vi "Inverse Kinematics Solution to Pod Setpoints.vi"(10 "actual theta":dbl, 11 "v + target":cluster{"velocity":dbl, "target theta":dbl}) -> (3 "new v + travel":cluster{"velocity":dbl, "travel angle":dbl})   [LabVIEW 2020]
doc: "takes the <b>current velocity</b> and <b>wanted target angle</b> to travel, finds the most efficient angle to travel, and outputs the <b>new velocity</b> and the <b>travel angle.</b>\n(used in inverse kinematics)"
uses:
  <vilib>/Analysis/coordinate.llb/Angle Units.ctl
  <vilib>/Analysis/coordinate.llb/Angle Range (Degree).ctl
  <vilib>/Analysis/coordinate.llb/Wrap Angle (scalar).vi
  <vilib>/Analysis/NI_AAL_Angle.lvlib
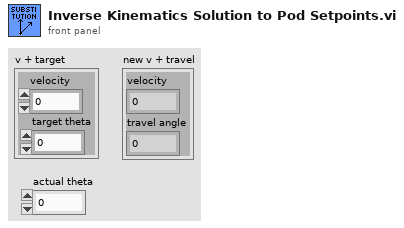
[diagram p1: front panel]
types:
  T1 = typedef "NI_AAL_Angle.lvlib/Angle Units.ctl" = i32
  T2 = typedef "NI_AAL_Angle.lvlib/Angle Range (Degree).ctl" = u16
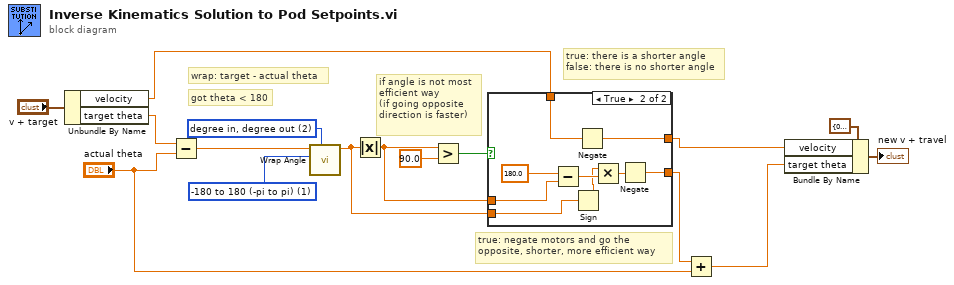
[diagram p0: block diagram]
diagram:
  w15 = T1 2 items=["radian in, radian out", "radian in, degree out", "degree in, degree out", "degree in, radian out"] ("angle units")
  w16 = T2 1 items=["none", "-180 to 180 (-pi to pi)", "0 to 360 (0 to 2pi)"] ("angle range")
  # "true: negate motors and go the\nopposite, shorter, more efficient way"
  # "if angle is not most\nefficient way\n(if going opposite \ndirection is faster)"
  # "true: there is a shorter angle\nfalse: there is no shorter angle"
  # "got theta < 180"
  # "wrap: target - actual theta"
  n1 = Unbundle By Name("v + target") -> ("velocity"=w11:dbl, "target theta"=w13:dbl)
  n2 = Subtract(x=w13, y="actual theta") -> (x-y=w12:dbl)
  n3 = call-poly <vilib>:"Wrap Angle.vi"("angle units"=w15, "angle range"=w16, "angle in"=w12) -> ("angle out"=w7:dbl)  [unwired: 7 in, 1 out]
  n4 = Absolute Value(x=w7) -> (abs(x)=w2:dbl)
  n5 = Greater?(x=w2, y=90.0) -> (0:w3:bool)
  n6 = case shown="True" w3 {
    tunnel: w11 -> [w18 w27]
    tunnel: [w18 w26] -> w10
    tunnel: w2 -> [_ w24]
    tunnel: [w17 w25] -> w5
    tunnel: w7 -> [w17 w21]
    frame False {
    }
    frame True {
      n7 = Subtract(x=180.0, y=w24) -> (x-y=w22:dbl)
      n8 = Sign(1:w21) -> (0:w20:dbl)
      n9 = Negate(x=w27) -> (-x=w26:dbl)
      n10 = Multiply(x=w20, y=w22) -> (x*y=w23:dbl)
      n11 = Negate(x=w23) -> (-x=w25:dbl)
    }
  }
  n12 = Add(x=w5, y="actual theta") -> (x+y=w4:dbl)
  n13 = Bundle By Name(cluster=cluster{"velocity":dbl, "target theta":dbl} {"velocity"=0.0, "target theta"=0.0}, "velocity"=w10, "target theta"=w4) -> (→"new v + travel":cluster{"velocity":dbl, "target theta":dbl})
